vi "PCF8574-NX-DM.vi"(0 "Input of PCF8574":T1={"Direction"=TRUE, "Address"=112, "Write Data"=255, "Compare"=0, "Compare Mask"=255} {"Compare Mask" format="%x"; "Compare" format="%x"; "Write Data" format="%x"; "Address" format="%x"}, 2 "NXT":T2={"error"={"status"=FALSE, "code"=0, "source"=""}, "address"="", "NXT #"=-1, "Show Error"=TRUE, "Connection"=4} {"Connection" items=["USB", "Bluetooth", "USB then Bluetooth", "Last Connection", "Preference"]}, 3 "Input Port":T3 items=["Port 1", "Port 2", "Port 3", "Port 4"]) -> (1 "Output of PCF8574":cluster{"Read Data":u8, bool}, 4 "NXT dup":T2={"error"={"status"=FALSE, "code"=0, "source"=""}, "address"="", "NXT #"=-1, "Show Error"=TRUE, "Connection"=4} {"Connection" items=["USB", "Bluetooth", "USB then Bluetooth", "Last Connection", "Preference"]})   [LabVIEW 2009]
uses:
  <vilib>/NXT/Block Support/NXT_InputPort.ctl
  <vilib>/NXT/Subs/LVHSConnector.ctl
  <vilib>/NXT/Block Support/HWPage.SensorType.ctl
  <vilib>/NXT/Block Support/HWPage.SensorMode.ctl
panel:
  out "Boolean":bool caption="Yes / No"
  out "Read Data":u8=255
  # "mindsensors.com\nCopyright (c) 2009 by mindsensors.com\nEmail: info (<at>) mindsensors (<dot>) com\n\nThis program is free software. You can redistribute it and/or modify\nit under the terms of the GNU General Public License as published by\nthe Free Software Foundation; version 3 of the License.\nRead the license at: http://www.gnu.org/licenses/gpl.txt"
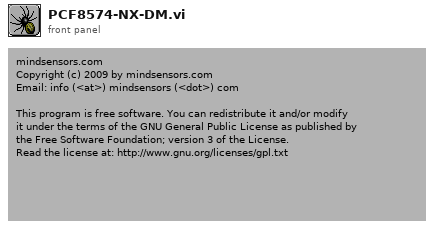
[diagram p1: front panel]
types:
  T1 = cluster{"Direction":bool, "Address":u8, "Write Data":u8, "Compare":u8, "Compare Mask":u8}
  T2 = typedef "LVHSConnector.ctl" = cluster{"error":errorcluster, "address":string, "NXT #":i32, "Show Error":bool, "Connection":u16}
  T3 = typedef "NXT_InputPort.ctl" = u8
  T4 = typedef "HWPage.SensorType.ctl" = u8
  T5 = typedef "HWPage.SensorMode.ctl" = u8
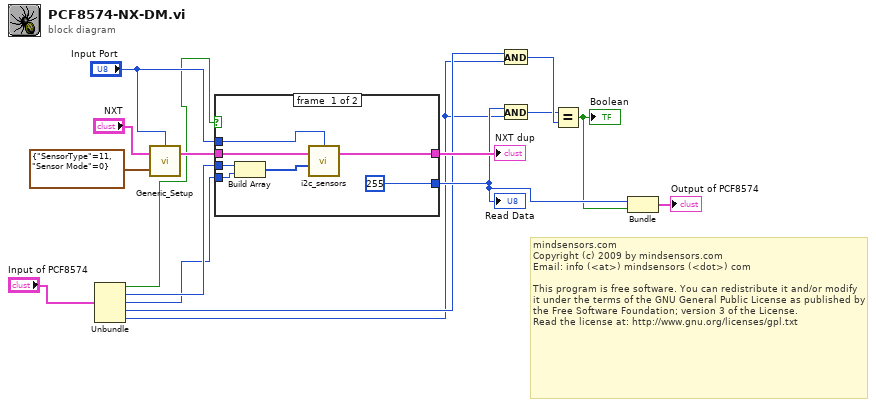
[diagram p0: block diagram]
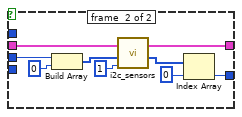
[diagram p2: hidden frame]
diagram:
  # "mindsensors.com\nCopyright (c) 2009 by mindsensors.com\nEmail: info (<at>) mindsensors (<dot>) com\n\nThis program is free software. You can redistribute it and/or modify\nit under the terms of the GNU General Public License as published by\nthe Free Software Foundation; version 3 of the License.\nRead the license at: http://www.gnu.org/licenses/gpl.txt"
  n1 = Unbundle("Input of PCF8574") -> ("Direction"=w5:bool, "Address"=w4:u8, "Write Data"=w3:u8, "Compare"=w2:u8, "Compare Mask"=w1:u8)
  n2 = call <vilib>:"Generic_Setup.vi"("Sensor Setup"=cluster{"SensorType":T4, "Sensor Mode":T5} {"SensorType"=11, "Sensor Mode"=0}, "NXT"="NXT", "Port"="Input Port") -> ("NXT"=w12:T2)  [unwired: 1 out]
  n3 = case shown="False" w5 {
    tunnel: "Input Port" -> [w22 _]
    tunnel: w4 -> [w20 w28]
    tunnel: w3 -> [w19 _]
    tunnel: [u8 255 w31] -> w9
    tunnel: w12 -> [w18 w25]
    tunnel: [w17 w24] -> w10
    frame #0 {
      n4 = Build Array(w20, w19) -> (w21:u8[])
      n5 = call <vilib>:"i2c_sensors.vi"("Bytes to Write"=w21, "NXT"=w18, "Port"=w22) -> ("NXT"=w17:T2)  [unwired: 2 in, 2 out]
    }
    frame #1 {
      n6 = Build Array(w28, u8 0 ("register")) -> (w29:u8[])
      n7 = call <vilib>:"i2c_sensors.vi"("Return Length"=u8 1 ("ReturnLength"), "Bytes to Write"=w29, "NXT"=w25) -> ("Bytes read"=w26:u8[], "NXT"=w24:T2)  [unwired: 2 in, 1 out]
      n8 = Index Array(array=w26, index=0) -> (element=w31:u8)
    }
  }
  "Read Data" <- w9
  "NXT dup" <- w10
  n9 = And(x=w2, y=w1) -> (x .and. y?=w16:u8)
  n10 = And(x=w9, y=w1) -> (x .and. y?=w15:u8)
  n11 = Equal?(x=w15, y=w16) -> (x = y?=w8:bool)
  "Boolean" <- w8
  n12 = Bundle(w9, w8) -> (→"Output of PCF8574":cluster{u8, bool})  [unwired: 1 in]
